vi "PBcard_init.vi"(1 "error in (no error)":errorcluster, 2 "Memory":bool=TRUE, 3 "Bytes/Word":u8=10, 4 "Select Board\nIndicator":i32) -> (0 "error out":errorcluster)   [LabVIEW 2013, in "PulseBlaster.lvlib"]
doc: "PBcard_INit: \nThis vi \n1) Selects the desired PB board\n2) resets the PB and sets some some reasonable defaults"
uses:
  PulseBlaster.lvlib
panel:
  # "External"
  # "Internal"
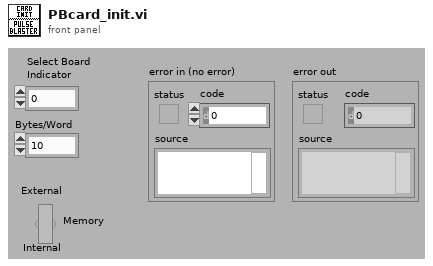
[diagram p1: front panel]
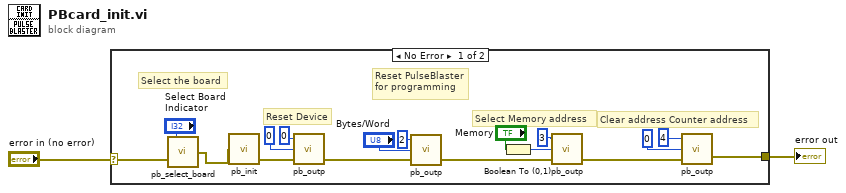
[diagram p0: block diagram]
diagram:
  n1 = case shown="No Error" "error in (no error)" {
    selector: "error in (no error)" -> [w3 w20]
    tunnel: [w15 w20] -> w1
    frame No Error {
      # "Select the board"
      # "Clear address Counter address"
      # "Select Memory address"
      # "Reset Device"
      # "Reset PulseBlaster\nfor programming"
      n2 = call "pb_select_board.vi"("error in (no error)"=w3, "Board to Address"="Select Board\nIndicator") -> ("error out"=w4:errorcluster)
      n3 = call "pb_init.vi"("error in (no error)"=w4) -> ("error out"=w19:errorcluster)
      n4 = call "pb_outp.vi"("error in (no error)"=w19, "8-bit data"=u8 0, "8-bit address offset"=u8 0) -> ("error out"=w18:errorcluster)
      n5 = call "pb_outp.vi"("error in (no error)"=w18, "8-bit data"="Bytes/Word", "8-bit address offset"=u8 2 ("Bytes per Word address")) -> ("error out"=w17:errorcluster)
      n6 = Boolean To (0,1)(Boolean="Memory") -> (0, 1=w9:i16)
      n7 = call "pb_outp.vi"("error in (no error)"=w17, "8-bit data"=w9, "8-bit address offset"=u8 3) -> ("error out"=w16:errorcluster)
      n8 = call "pb_outp.vi"("error in (no error)"=w16, "8-bit data"=u8 0, "8-bit address offset"=u8 4) -> ("error out"=w15:errorcluster)
    }
    frame Error {
    }
  }
  "error out" <- w1
